vi "Send Message.vi"(7 "Message Type":T1, 11 "Message":string) -> ()   [LabVIEW 2014]
uses:
  Controls/Telemetry Header.ctl
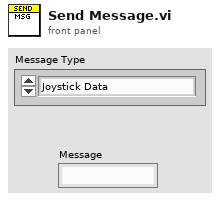
[diagram p1: front panel]
types:
  T1 = typedef "Telemetry Header.ctl" = enum16{"Joystick Data", "Position Data"}
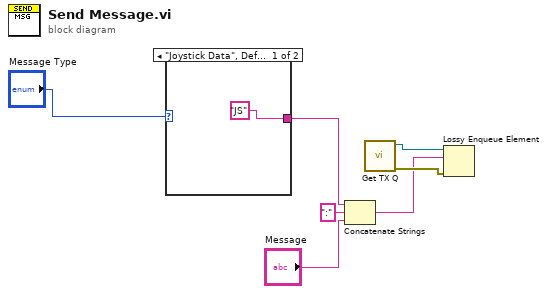
[diagram p0: block diagram]
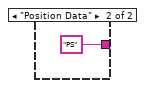
[diagram p2: hidden frame]
diagram:
  n1 = case shown="\"Joystick Data\", Default" "Message Type" {
    tunnel: ["JS" "PS"] -> w1
    frame "Joystick Data", Default {
    }
    frame "Position Data" {
    }
  }
  n2 = Concatenate Strings(w1, ":" ("string"), "Message") -> (w4:string)
  n3 = call "Get TX Q.vi"() -> ("error out"=w6:errorcluster, "TX Q"=w7:refnum<queue>)  [unwired: 10 in]
  n4 = Lossy Enqueue Element(queue=w7, element=w4, error in (no error)=w6) -> ()  [unwired: 4 out]
